vi "__SISBias_init.vi"(7 "Bias_LO_equip":T1={"Node address"=19, "CAN Interface"="CAN0", "Cartridge band"=10, "Slave Node in"={"Address"=19, "Serial Number"=[16, 71, 55, 76, 1, 8, 0, -15]}, "ObjHandle out"=93192256, "POL"=0, "sb"=1, "GPIB_SM (SIS S,V)"="24", "GPIB_DMM (SIS I)"="22", "GPIB_SM (MAG I) "="25", "GPIB_SG(LO)"="19", "GPIB_PW (PAMP) "="6", "GPIB_TMP1(8ch)"="12", "GPIB_TMP2(2ch)  "="13", "WCA_avg"=10, "Rsen"=10.0, "BiasModule"=1, "LOModule "=5, "WCA_LO_FREQ_SET"={"YTO Low freq. [GHz]"=14.42, "YTO High freq. [GHz]"=17.7, "Kvco"=1, "Lock Pol."=0, "SET LO FREQ"=96.22222, "Multiplier"=6.0, "YTO (HEX)"=2014, "YTO coarse( FREQ)"=16.033167, "NULL PLL INTEGRATOR"=FALSE}, "Res for"=0} {"Res for" items=["none", "series res", "parallel res"]; "WCA_LO_FREQ_SET"."YTO coarse( FREQ)" min=25 max=150 step=0.0001 format="%.3f"; "WCA_LO_FREQ_SET"."Multiplier" min=3 max=6 step=3; "WCA_LO_FREQ_SET"."SET LO FREQ" min=25 max=150 step=0.0001 format="%.3f"; "WCA_LO_FREQ_SET"."Lock Pol." items=["Lower", "Upper"]; "WCA_LO_FREQ_SET"."Kvco" items=["7.5MHz/V", "15MHz/V"]; "WCA_LO_FREQ_SET"."YTO High freq. [GHz]" format="%.3f"; "WCA_LO_FREQ_SET"."YTO Low freq. [GHz]" format="%.3f"; "BiasModule" items=["B10Lab Bias"=0, "WCA BiasModule"=1, "none"=99]; "Slave Node in"."Serial Number" format="%.0x"; "Slave Node in"."Address" format="%.0x"; "Cartridge band" max=10 step=1; "Node address" format="%.0x"}) -> (0 "error out":errorcluster caption="エラー出力", 1 "Detected CAN Nodes.":string, 3 "Bias_LO_equip 2":T1={"Node address"=19, "CAN Interface"="CAN0", "Cartridge band"=10, "Slave Node in"={"Address"=19, "Serial Number"=[16, 71, 55, 76, 1, 8, 0, -15]}, "ObjHandle out"=93192256, "POL"=0, "sb"=1, "GPIB_SM (SIS S,V)"="24", "GPIB_DMM (SIS I)"="22", "GPIB_SM (MAG I) "="25", "GPIB_SG(LO)"="19", "GPIB_PW (PAMP) "="6", "GPIB_TMP1(8ch)"="12", "GPIB_TMP2(2ch)  "="13", "WCA_avg"=10, "Rsen"=10.0, "BiasModule"=1, "LOModule "=5, "WCA_LO_FREQ_SET"={"YTO Low freq. [GHz]"=14.42, "YTO High freq. [GHz]"=17.7, "Kvco"=1, "Lock Pol."=0, "SET LO FREQ"=96.22222, "Multiplier"=6.0, "YTO (HEX)"=2014, "YTO coarse( FREQ)"=16.033167, "NULL PLL INTEGRATOR"=FALSE}, "Res for"=0} {"Res for" items=["none", "series res", "parallel res"]; "WCA_LO_FREQ_SET"."YTO coarse( FREQ)" min=25 max=150 step=0.0001 format="%.3f"; "WCA_LO_FREQ_SET"."Multiplier" min=3 max=6 step=3; "WCA_LO_FREQ_SET"."SET LO FREQ" min=25 max=150 step=0.0001 format="%.3f"; "WCA_LO_FREQ_SET"."Lock Pol." items=["Lower", "Upper"]; "WCA_LO_FREQ_SET"."Kvco" items=["7.5MHz/V", "15MHz/V"]; "WCA_LO_FREQ_SET"."YTO High freq. [GHz]" format="%.3f"; "WCA_LO_FREQ_SET"."YTO Low freq. [GHz]" format="%.3f"; "BiasModule" items=["B10Lab Bias"=0, "WCA BiasModule"=1, "none"=99]; "Slave Node in"."Serial Number" format="%.0x"; "Slave Node in"."Address" format="%.0x"; "Cartridge band" max=10 step=1; "Node address" format="%.0x"})   [LabVIEW 2017]
panel:
  # "LO freq. [GHz]"
  # "YTO LOW\n/High Freq."
  # "ZERO Intgrtr"
  # "Node Address"
  # "Serial Number"
  # "LO freq. [GHz]"
  # "YTO LOW\n/High Freq."
  # "ZERO Intgrtr"
  # "Node Address"
  # "Serial Number"
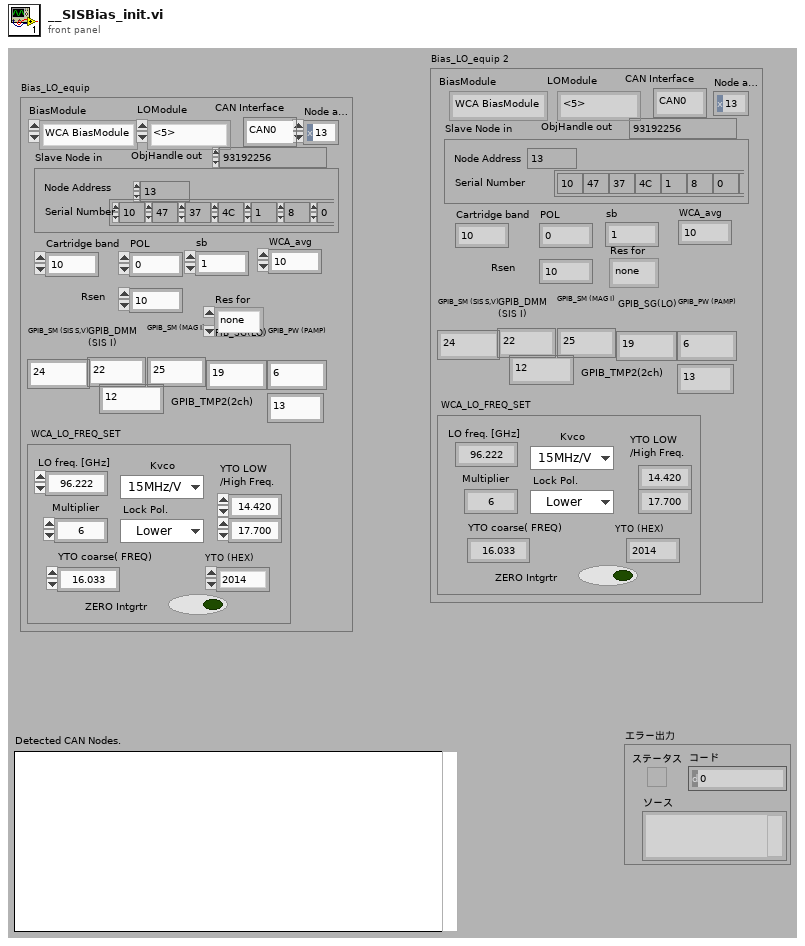
[diagram p1: front panel]
types:
  T1 = cluster{"Node address":u16, "CAN Interface":string, "Cartridge band":u32, "Slave Node in":cluster{"Address":i16, "Serial Number":i8[]}, "ObjHandle out":u32, "POL":u32, "sb":u32, "GPIB_SM (SIS S,V)":string, "GPIB_DMM (SIS I)":string, "GPIB_SM (MAG I) ":string, "GPIB_SG(LO)":string, "GPIB_PW (PAMP) ":string, "GPIB_TMP1(8ch)":string, "GPIB_TMP2(2ch)  ":string, "WCA_avg":i32, "Rsen":dbl, "BiasModule":u16, "LOModule ":u16, "WCA_LO_FREQ_SET":cluster{"YTO Low freq. [GHz]":sgl, "YTO High freq. [GHz]":sgl, "Kvco":u16, "Lock Pol.":u16, "SET LO FREQ":sgl, "Multiplier":sgl, "YTO (HEX)":u16, "YTO coarse( FREQ)":sgl, "NULL PLL INTEGRATOR":bool}, "Res for":u16}
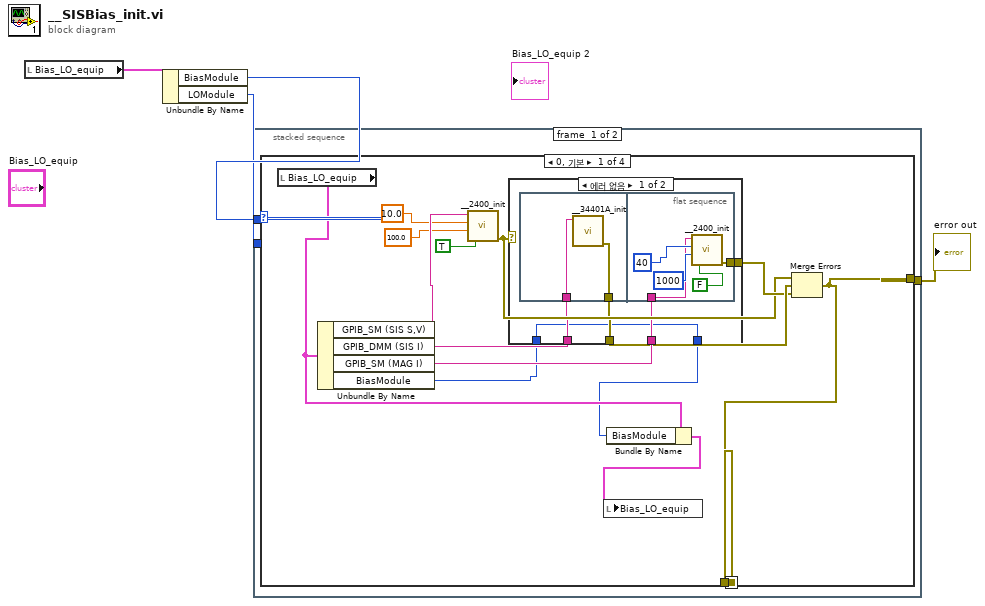
[diagram p0: block diagram]
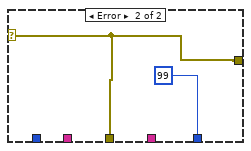
[diagram p2: hidden frame]
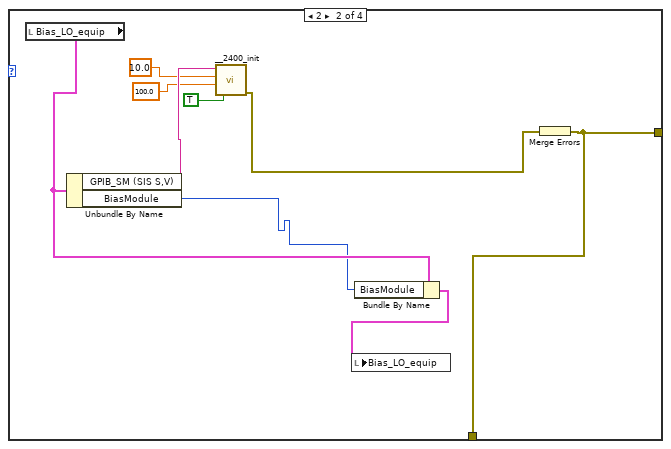
[diagram p3: hidden frame]
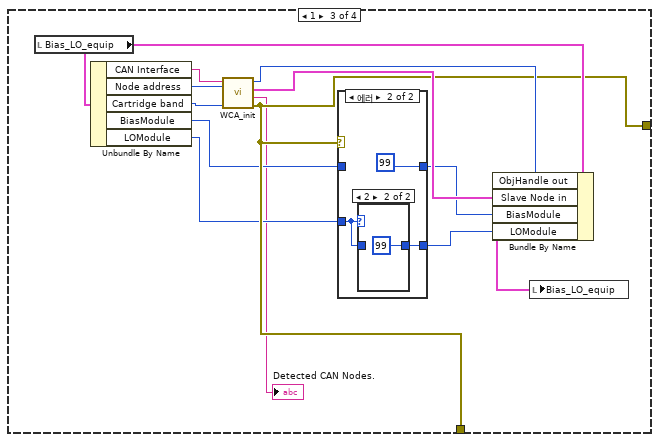
[diagram p4: hidden frame]
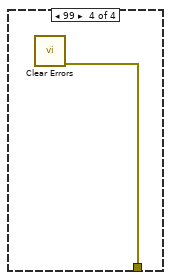
[diagram p7: hidden frame]
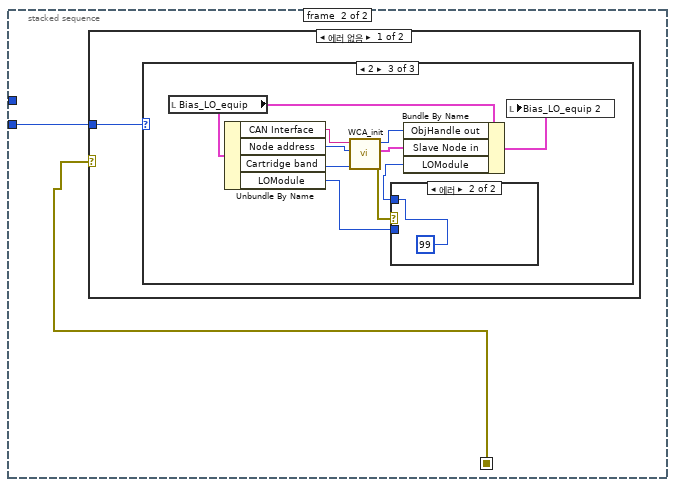
[diagram p8: hidden frame]
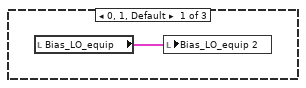
[diagram p9: hidden frame]
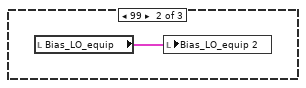
[diagram p10: hidden frame]
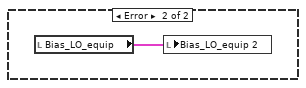
[diagram p12: hidden frame]
diagram:
  n1 = local read "Bias_LO_equip"() -> (w3:T1)
  n2 = Unbundle By Name(w3) -> ("BiasModule"=w2:u16, "LOModule"=w1:u16)
  n3 = stacked-sequence {
    seq-local: [w5 _] -> [_ w66]
    tunnel: [w7 _] -> w4
    tunnel: w2 -> [w6 _]
    tunnel: w1 -> [_ w67]
    frame #0 {
      n4 = case shown="0, 기본" w6 {
        tunnel: [w17 w44 w50 _] -> w7
        tunnel: [w17 w44 w50 w65] -> w5
        frame 0, Default {
          n5 = local read "Bias_LO_equip"() -> (w11:T1)
          n6 = Unbundle By Name(w11) -> ("GPIB_SM (SIS S,V)"=w15:string, "GPIB_DMM (SIS I)"=w21:string, "GPIB_SM (MAG I)"=w20:string, "BiasModule"=w9:u16)
          n7 = call "__2400_init.vi"("‚SW"=TRUE, "volt_range(mV)"=100.0, "curr_range(mA)"=10.0, "GPIB"=w15) -> ("error out"=w14:errorcluster)  [unwired: 3 in]
          n8 = case shown="에러 없음" w14 {
            selector: w14 -> [_ w35]
            tunnel: w21 -> [w26 _]
            tunnel: w20 -> [w25 _]
            tunnel: [w24 w35] -> w19
            tunnel: [w23 w35] -> w18
            tunnel: [w22 99] -> w10
            tunnel: w9 -> [w22 _]
            frame No Error {
              n9 = flat-sequence {
                tunnel: w26 -> [w28]
                tunnel: [w27] -> w24
                tunnel: w25 -> [w30]
                tunnel: [w29] -> w23
                frame #0 {
                  n10 = call "__34401A_init.vi"("GPIB"=w28) -> ("error out"=w27:errorcluster)  [unwired: 6 in]
                }
                frame #1 {
                  n11 = call "__2400_init.vi"("‚SW"=FALSE, "volt_range(mV)"=1000, "curr_range(mA)"=40, "GPIB"=w30) -> ("error out"=w29:errorcluster)  [unwired: 3 in]
                }
              }
            }
            frame Error {
            }
          }
          n12 = Bundle By Name(cluster=w11, "BiasModule"=w10) -> (w8:T1)
          n13 = local write "Bias_LO_equip"(w8) -> ()
          n14 = Merge Errors(w14, w19, w18) -> (w17:errorcluster)
        }
        frame 2 {
          n15 = local read "Bias_LO_equip"() -> (w38:T1)
          n16 = Unbundle By Name(w38) -> ("GPIB_SM (SIS S,V)"=w42:string, "BiasModule"=w36:u16)
          n17 = call "__2400_init.vi"("‚SW"=TRUE, "volt_range(mV)"=100.0, "curr_range(mA)"=10.0, "GPIB"=w42) -> ("error out"=w41:errorcluster)  [unwired: 3 in]
          n18 = Bundle By Name(cluster=w38, "BiasModule"=w36) -> (w37:T1)
          n19 = local write "Bias_LO_equip"(w37) -> ()
          n20 = Merge Errors(w41) -> (w44:errorcluster)
        }
        frame 1 {
          n21 = local read "Bias_LO_equip"() -> (w52:T1)
          n22 = Unbundle By Name(w52) -> ("CAN Interface"=w55:string, "Node address"=w54:u16, "Cartridge band"=w53:u32, "BiasModule"=w49:u16, "LOModule"=w47:u16)
          n23 = call "WCA_init.vi"("Cartridge band"=w53, "Node address"=w54, "CAN Interface"=w55) -> ("error out 2"=w50:errorcluster, "Detected CAN Nodes."=→"Detected CAN Nodes.":string, "Slave Node in"=w56:cluster{"Address":i16, "Serial Number":i8[]}, "ObjHandle out"=w57:u32)  [unwired: 4 in, 1 out]
          n24 = case shown="에러" w50 {
            tunnel: [w59 99] -> w48
            tunnel: w49 -> [w59 _]
            tunnel: w47 -> [w58 w60]
            tunnel: [w58 w61] -> w46
            frame No Error {
            }
            frame Error {
              n25 = case shown="2" w60 {
                tunnel: [w63 99] -> w61
                tunnel: w60 -> [w63 _]
                frame 0, Default {
                }
                frame 2 {
                }
              }
            }
          }
          n26 = Bundle By Name(cluster=w52, "ObjHandle out"=w57, "Slave Node in"=w56, "BiasModule"=w48, "LOModule"=w46) -> (w51:T1)
          n27 = local write "Bias_LO_equip"(w51) -> ()
        }
        frame 99 {
          n28 = call <vilib>:"Clear Errors.vi"() -> ("error out"=w65:errorcluster)  [unwired: 6 in, 1 out]
        }
      }
    }
    frame #1 {
      n29 = case shown="에러 없음" w66 {
        tunnel: w67 -> [w68 _]
        frame No Error {
          n30 = case shown="2" w68 {
            frame 0, 1, Default {
              n31 = local read "Bias_LO_equip"() -> (w69:T1)
              n32 = local write "Bias_LO_equip 2"(w69) -> ()
            }
            frame 99 {
              n33 = local read "Bias_LO_equip"() -> (w70:T1)
              n34 = local write "Bias_LO_equip 2"(w70) -> ()
            }
            frame 2 {
              n35 = local read "Bias_LO_equip"() -> (w75:T1)
              n36 = Unbundle By Name(w75) -> ("CAN Interface"=w78:string, "Node address"=w77:u16, "Cartridge band"=w76:u32, "LOModule"=w71:u16)
              n37 = call "WCA_init.vi"("Cartridge band"=w76, "Node address"=w77, "CAN Interface"=w78) -> ("error out 2"=w73:errorcluster, "Slave Node in"=w79:cluster{"Address":i16, "Serial Number":i8[]}, "ObjHandle out"=w80:u32)  [unwired: 4 in, 2 out]
              n38 = case shown="에러" w73 {
                tunnel: [w81 99] -> w72
                tunnel: w71 -> [w81 _]
                frame No Error {
                }
                frame Error {
                }
              }
              n39 = Bundle By Name(cluster=w75, "ObjHandle out"=w80, "Slave Node in"=w79, "LOModule"=w72) -> (w74:T1)
              n40 = local write "Bias_LO_equip 2"(w74) -> ()
            }
          }
        }
        frame Error {
          n41 = local read "Bias_LO_equip"() -> (w83:T1)
          n42 = local write "Bias_LO_equip 2"(w83) -> ()
        }
      }
    }
  }
  "error out" <- w4
